vi "AB_RW_Project_WebService_Info.vi"(7 "action":T2, 8 "error in (no error)":errorcluster, 10 "webServiceInfo in":T1, 11 "Object In":T3) -> (0 "error out":errorcluster, 2 "webServiceInfo out":T1, 3 "Object Out":T3)   [LabVIEW 2020]
uses:
  <resource>/Framework/Providers/API/ItemRef.ctl
  <vilib>/AppBuilder/RW_Project/AB_RW_Project_PropBag_Action.ctl
  <vilib>/AppBuilder/RW_Project/AB_RW_Project_WebService_Data.ctl
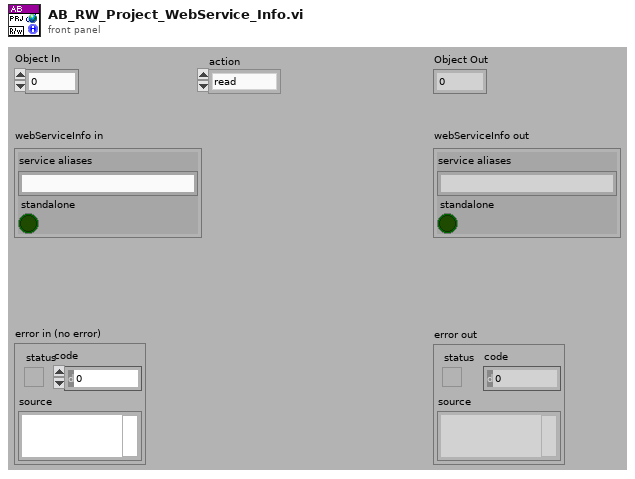
[diagram p1: front panel]
types:
  T1 = typedef "AB_RW_Project_WebService_Data.ctl" = cluster{"service aliases":string, "standalone":bool}
  T2 = typedef "AB_RW_Project_PropBag_Action.ctl" = enum16{"read", "write", "clear", "readPrevious", "writePrevious", "clearPrevious"}
  T3 = typedef "ItemRef.ctl" = u64
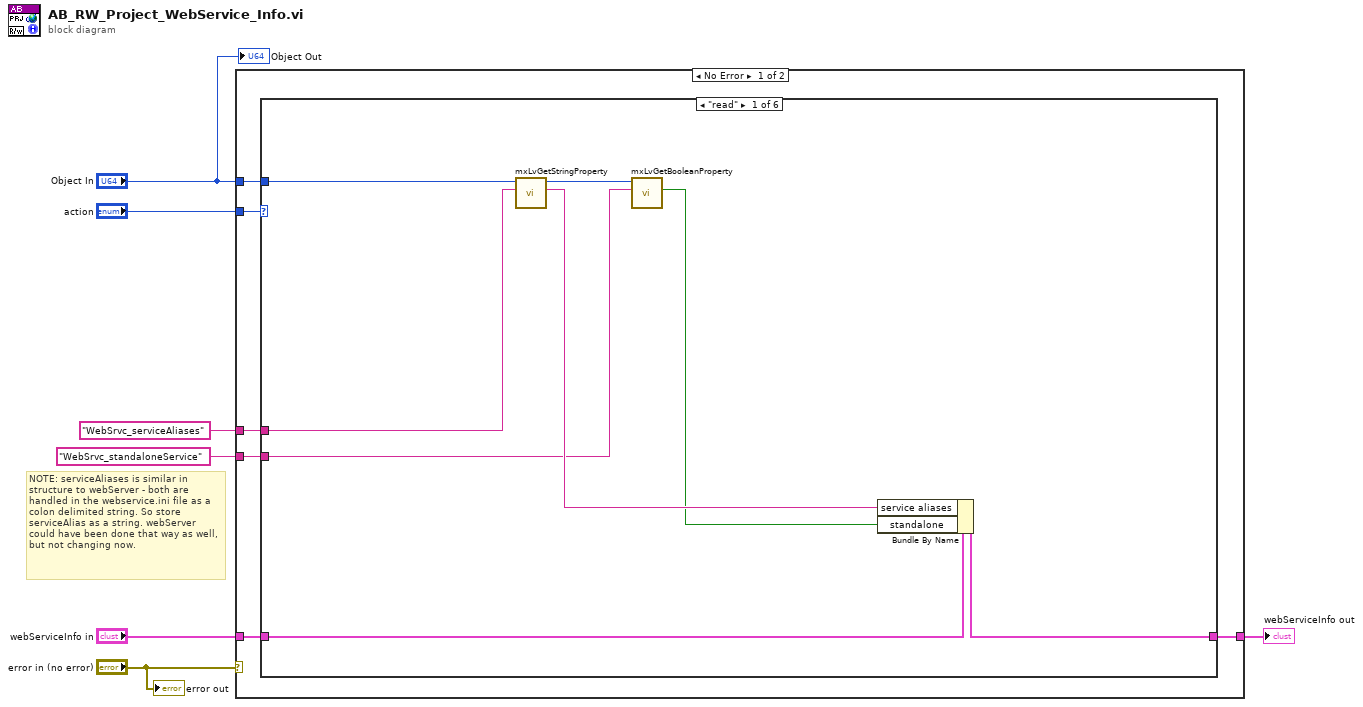
[diagram p0: block diagram]
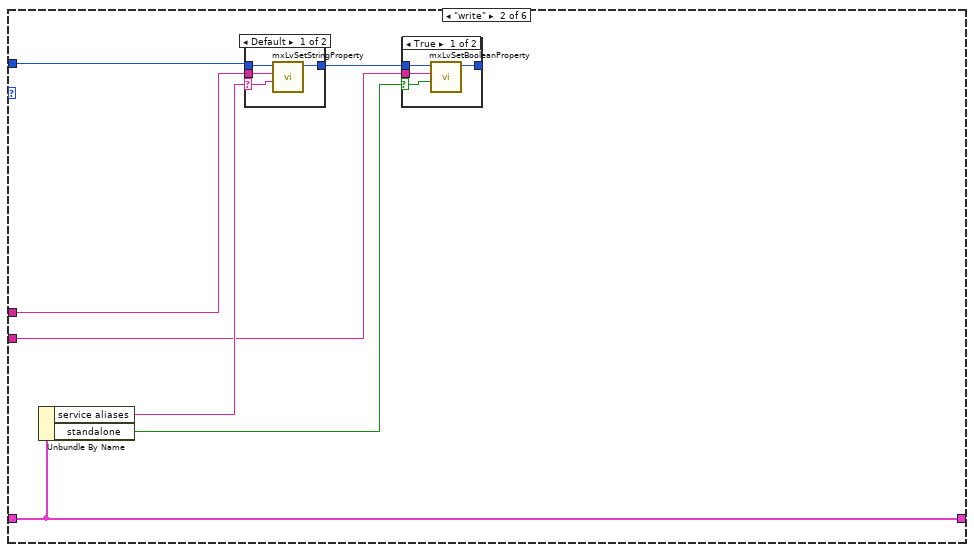
[diagram p2: hidden frame]
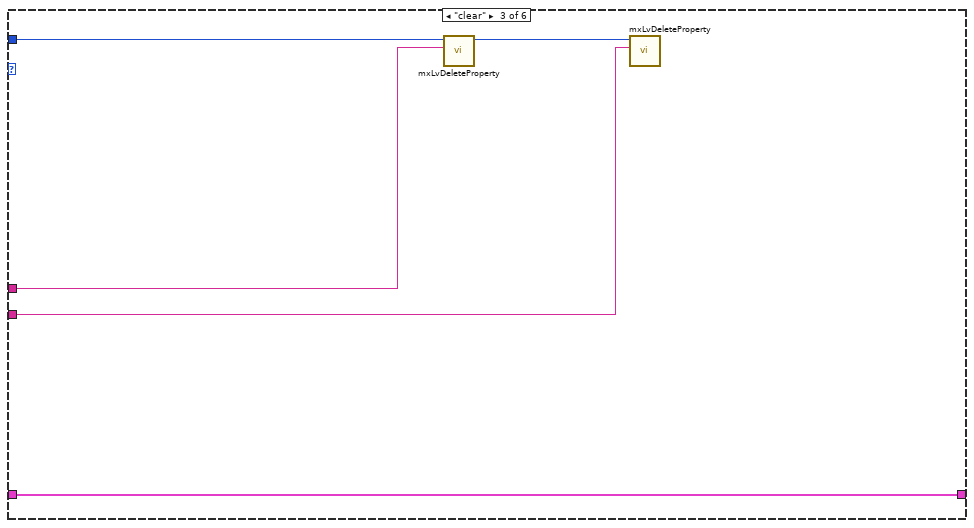
[diagram p5: hidden frame]
diagram:
  # "NOTE: serviceAliases is similar in structure to webServer - both are handled in the webservice.ini file as a colon delimited string. So store serviceAlias as a string. webServer could have been done that way as well, but not changing now."
  n1 = case shown="No Error" "error in (no error)" {
    tunnel: "Object In" -> [w13 _]
    tunnel: [w10 _] -> w3
    tunnel: "webServiceInfo in" -> [w12 _]
    tunnel: "action" -> [w11 _]
    tunnel: "WebSrvc_serviceAliases" ("Tag") -> [w9 _]
    tunnel: "WebSrvc_standaloneService" ("Tag") -> [w8 _]
    frame No Error {
      n2 = case shown="\"read\"" w11 {
        tunnel: w13 -> [w17 w27 w41 _ _ _]
        tunnel: w12 -> [w20 w28 w43 w44 w45 w46]
        tunnel: [w21 w28 w43 w44 w45 w46] -> w10
        tunnel: w9 -> [w19 w26 w40 _ _ _]
        tunnel: w8 -> [w15 w22 w39 _ _ _]
        frame "read" {
          n3 = call <resource>:"mxLvGetStringProperty.vi"("Tag"=w19, "Item"=w17) -> ("Value"=w18:string, "Item"=w16:T3)  [unwired: 1 in, 7 out]
          n4 = call <resource>:"mxLvGetBooleanProperty.vi"("Tag"=w15, "Item"=w16) -> ("Value"=w14:bool)  [unwired: 1 in, 8 out]
          n5 = Bundle By Name(cluster=w20, "service aliases"=w18, "standalone"=w14) -> (w21:T1)
        }
        frame "write" {
          n6 = Unbundle By Name(w28) -> ("service aliases"=w25:string, "standalone"=w23:bool)
          n7 = case shown="Default" w25 {
            selector: w25 -> [w35 _]
            tunnel: w27 -> [w37 w38]
            tunnel: w26 -> [w36 _]
            tunnel: [w34 w38] -> w24
            frame Default {
              n8 = call <resource>:"mxLvSetStringProperty.vi"("Value (\"\")"=w35, "Tag"=w36, "Item"=w37) -> ("Item"=w34:T3)  [unwired: 2 in, 6 out]
            }
            frame "" {
            }
          }
          n9 = case shown="True" w23 {
            selector: w23 -> [w31 _]
            tunnel: w24 -> [w32 w33]
            tunnel: w22 -> [w30 _]
            tunnel: [w29 w33] -> _
            frame True {
              n10 = call <resource>:"mxLvSetBooleanProperty.vi"("Value (F)"=w31, "Tag"=w30, "Item"=w32) -> ("Item"=w29:T3)  [unwired: 2 in, 6 out]
            }
            frame False {
            }
          }
        }
        frame "clear" {
          n11 = call <resource>:"mxLvDeleteProperty.vi"("Tag"=w40, "Item"=w41) -> ("Item"=w42:T3)  [unwired: 1 in, 8 out]
          n12 = call <resource>:"mxLvDeleteProperty.vi"("Tag"=w39, "Item"=w42) -> ()  [unwired: 1 in, 9 out]
        }
        frame "readPrevious" {
        }
        frame "writePrevious" {
        }
        frame "clearPrevious" {
        }
      }
    }
    frame Error {
    }
  }
  "webServiceInfo out" <- w3
  "Object Out" <- "Object In"
  "error out" <- "error in (no error)"
